vi "IncrementIndex.vi"(8 "Increment?":bool, 11 "IndexIn":i32) -> (3 "IndexOut":i32)   [LabVIEW 2015]
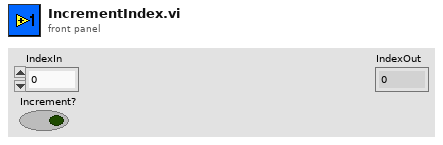
[diagram p1: front panel]
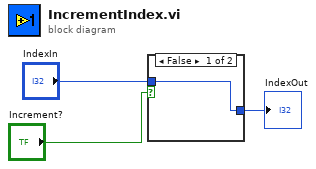
[diagram p0: block diagram]
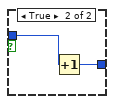
[diagram p2: hidden frame]
diagram:
  n1 = case shown="False" "Increment?" {
    tunnel: "IndexIn" -> [w4 w5]
    tunnel: [w4 w6] -> w1
    frame False {
    }
    frame True {
      n2 = Increment(x=w5) -> (x+1=w6:i32)
    }
  }
  "IndexOut" <- w1
